vi "Changer.vi"(0 "toChanger":T1(array[cluster]), 1 "out":u8[](array[numeric]), 2 "in":u8[](array[numeric])) -> ()   [LabVIEW 2010]
panel:
  out "error out":errorcluster
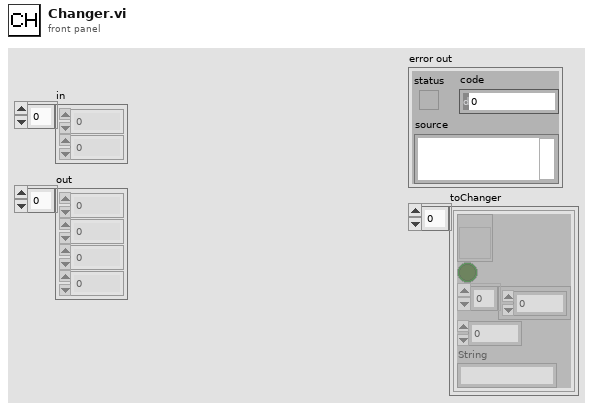
[diagram p1: front panel]
types:
  T1 = cluster{refnum<vi>, bool, i32[], i32, "String":string}[]
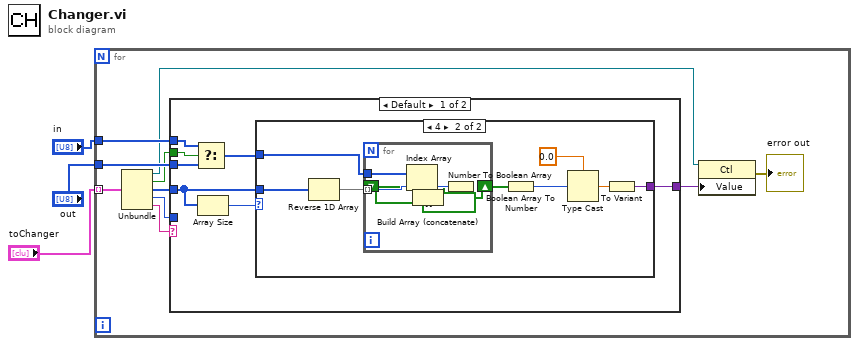
[diagram p0: block diagram]
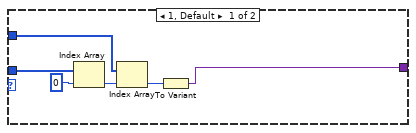
[diagram p2: hidden frame]
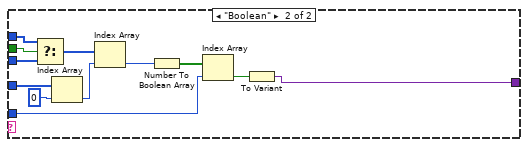
[diagram p3: hidden frame]
diagram:
  n1 = for {
    tunnel: "out" -> [w13]
    tunnel: "toChanger" -> [w12] mode=indexing
    tunnel: "in" -> [w10]
    n2 = Unbundle(w12) -> (w6:refnum<vi>, w9:bool, w8:i32[], w11:i32, "String"=w7:string)
    n3 = case shown="Default" w7 {
      tunnel: w13 -> [w20 w52]
      tunnel: w11 -> [_ w48]
      tunnel: w10 -> [w19 w47]
      tunnel: w9 -> [w18 w46]
      tunnel: w8 -> [w16 w45]
      tunnel: [w14 w42] -> w4
      frame Default {
        n4 = Select(t=w19, s=w18, f=w20) -> (s? t:f=w15:u8[])
        n5 = Array Size(array=w16) -> (size(s)=w17:i32)
        n6 = case shown="4" w17 {
          tunnel: w16 -> [w26 w33]
          tunnel: w15 -> [w24 w35]
          tunnel: [w21 w32] -> w14
          frame 1, Default {
            n7 = Index Array(array=w26, index=0) -> (element=w23:i32)
            n8 = Index Array(array=w24, index=w23) -> (element=w22:u8)
            n9 = To Variant(anything=w22) -> (Variant=w21:variant)
          }
          frame 4 {
            n10 = Reverse 1D Array(array=w33) -> (reversed array=w34:i32[])
            n11 = for {
              tunnel: w35 -> [w41]
              tunnel: w34 -> [w40] mode=indexing
              shift-right: [w36] -> w30
              shift-left: bool[] [] ("Boolean array") -> [w37]
              n12 = Index Array(array=w41, index=w40) -> (element=w39:u8)
              n13 = Number To Boolean Array(number=w39) -> (Boolean array=w38:bool[])
              n14 = Build Array (concatenate)(w37, w38) -> (w36:bool[])
            }
            n15 = Boolean Array To Number(Boolean array=w30) -> (number=w31:u32)
            n16 = Type Cast(type=sgl 0.0, x=w31) -> (*(type *) &x=w28:sgl)
            n17 = To Variant(anything=w28) -> (Variant=w32:variant)
          }
        }
      }
      frame "Boolean" {
        n18 = Select(t=w47, s=w46, f=w52) -> (s? t:f=w51:u8[])
        n19 = Index Array(array=w45, index=0) -> (element=w43:i32)
        n20 = Index Array(array=w51, index=w43) -> (element=w50:u8)
        n21 = Number To Boolean Array(number=w50) -> (Boolean array=w53:bool[])
        n22 = Index Array(array=w53, index=w48) -> (element=w49:bool)
        n23 = To Variant(anything=w49) -> (Variant=w42:variant)
      }
    }
    n24 = property on="Property Node" class="Ctl"(reference=w6, "Value"=w4) -> (error out=→"error out":errorcluster)  [unwired: 1 in, 1 out]
  }
